vi "LDA_High_Convert_New.vi"(1 "dimensions":enum16{"1D", "2D"}(ring)=enum."2D", 2 "Create Sync Index":bool) -> (3 "LDA data":dbl[][](array[numeric]) format="%.3f", 5 "Diagnostic info":string[][](table), 6 "Sync Index":i32[](array[numeric]))   [LabVIEW 2017]
uses:
  BSA_Type.ctl
  Globals/LDA_meas_global_1.vi
  Globals/Plug_in_data_global.vi
  Globals/Meas_global.vi
  Globals/Preference_global.vi
  Globals/LDA_meas_global_2.vi
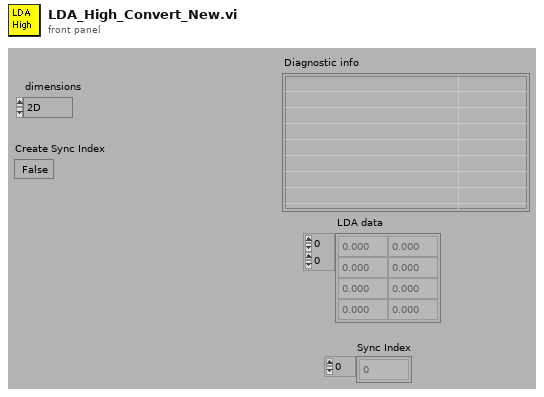
[diagram p1: front panel]
types:
  T1 = typedef "BSA_Type.ctl" = enum16{"57N11", "BSA F60"}
  T2 = enum16{"Velocity", "Transit time", "Arrival time"}[]
  T3 = typedef "Analysis_info_cluster.ctl" = cluster{"Colour":u32, "Inst type":T4, "Inst name":string, "Symbol":string, "Code name":string, "Extra Info":string, "Inst Array":T5, "Extra Titles":string[], "Extra Values":string[], "U":dbl, "u^2":dbl, "u^3":dbl, "u^4":dbl, "Skew_u":dbl, "Kurt_u":dbl, "Sd Error in Mean":dbl, "% u'/U":dbl, "X":dbl, "Y":dbl, "Z":dbl, "Timescale integral Estimate":dbl, "Sd Error in Variance":dbl, "Calib File":path, "Calib Constants":dbl[], "Output Position":bool, "Full Stats":bool, "Av Sampling Rate":dbl, "Av No of Samples":dbl, "Total Meas Time (s)":dbl, "ADAM Ch Name":string, "Max value":dbl, "Min value":dbl, "Sync Delay Time (s)":dbl, "Device ID":string, "Req Sample Rate Hz":dbl}
  T4 = typedef "Inst_type.ctl" = enum16{"Propeller anemometer", "Raw voltage", "Pressure Transducer", "Pitot-static tube", "Preston tube", "Hot wire", "Cross wire 1", "Cross wire 2", "Generic Linear", "Generic Polynomial", "Generic BackPoly", "Fast FID", "Thermocouple", "Cold wire", "Pulsed Wire", "LDA Vel", "LDA Tran time", "LDA Arr time", "Microphone"}
  T5 = typedef "Instrument_Array.ctl" = enum16{"PWA", "LDA", "Analogue"}
  T6 = typedef "Time_Trace_Cluster.ctl" = cluster{"Weighting":dbl[], "Time (s)":dbl[], "Voltage":dbl[], "Eng Values":dbl[]}
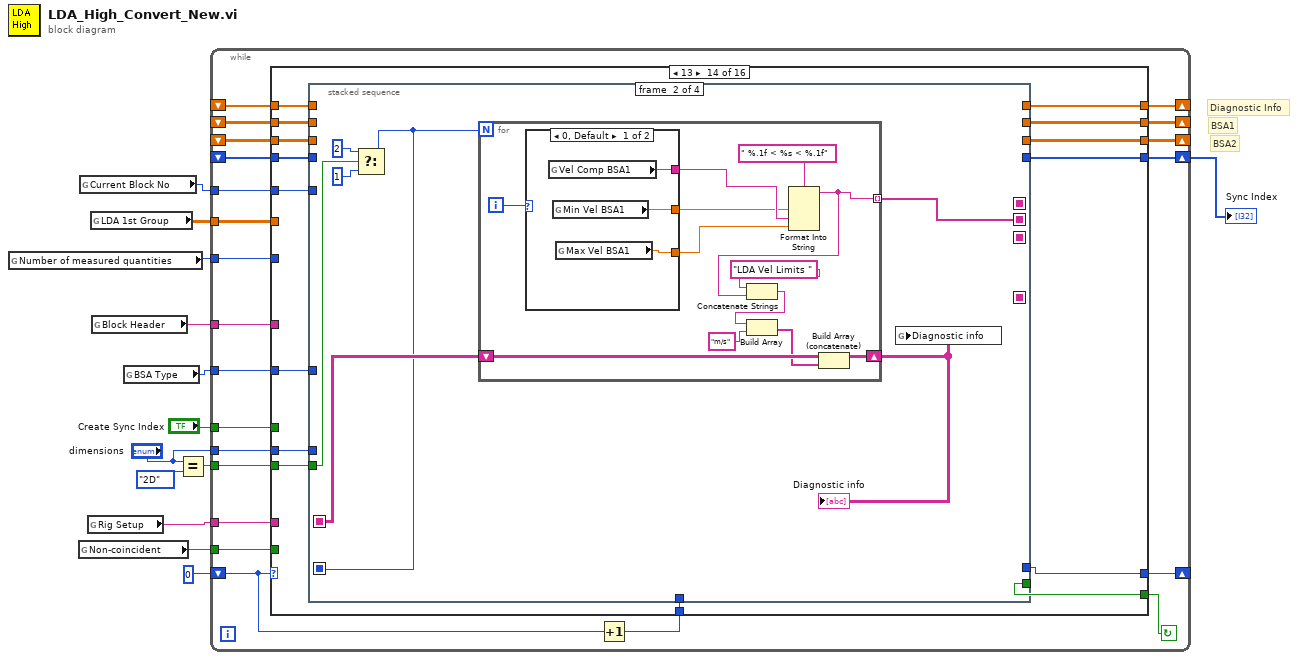
[diagram p0: block diagram]
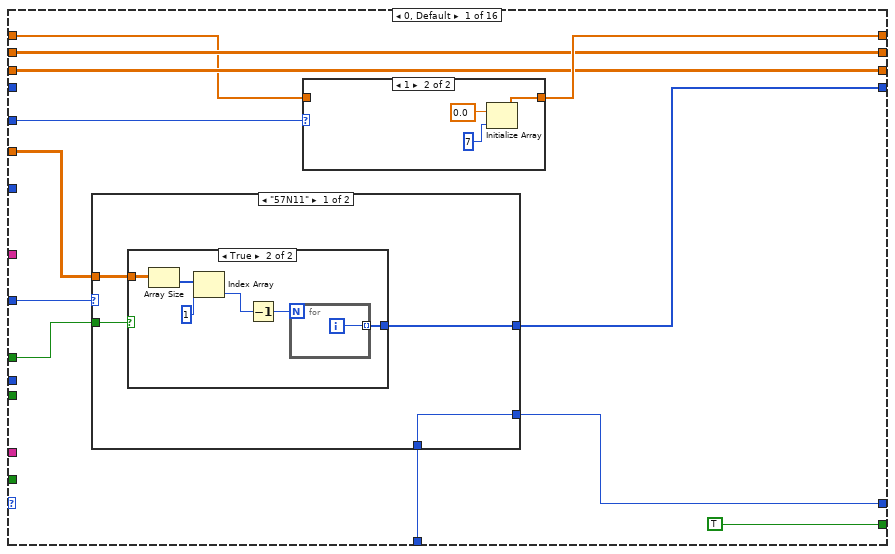
[diagram p2: hidden frame]
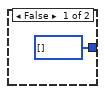
[diagram p4: hidden frame]
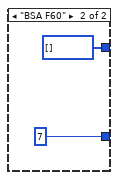
[diagram p5: hidden frame]
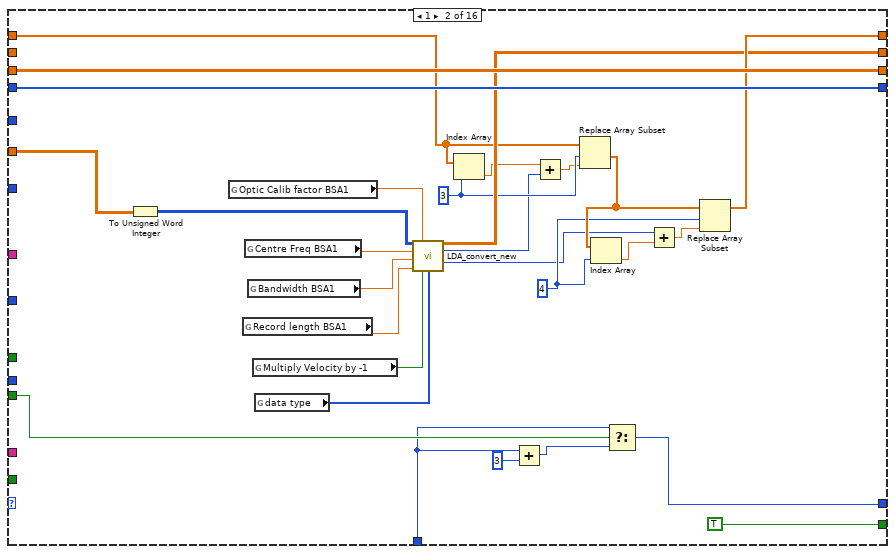
[diagram p6: hidden frame]
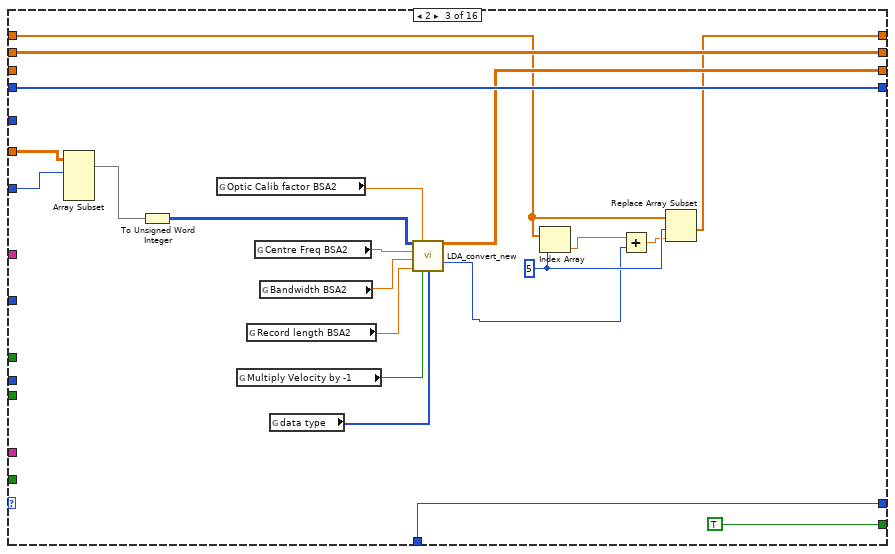
[diagram p7: hidden frame]
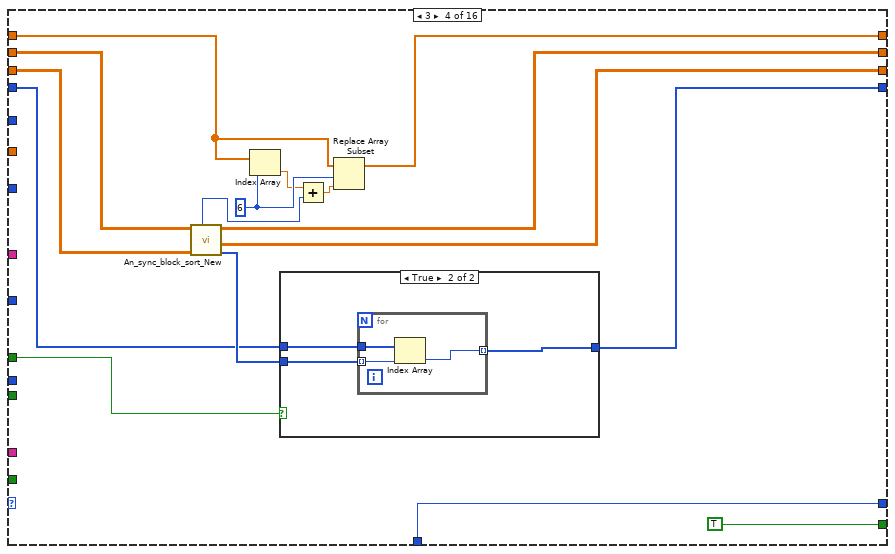
[diagram p8: hidden frame]
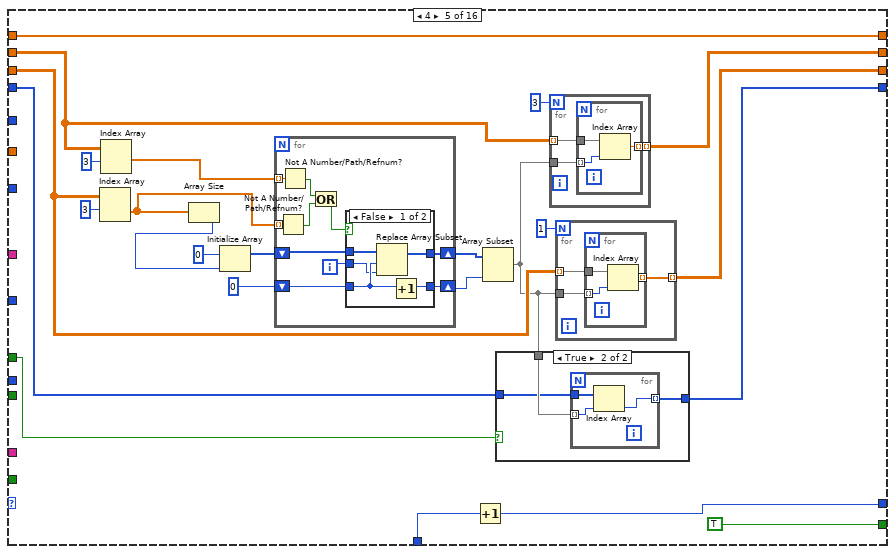
[diagram p10: hidden frame]
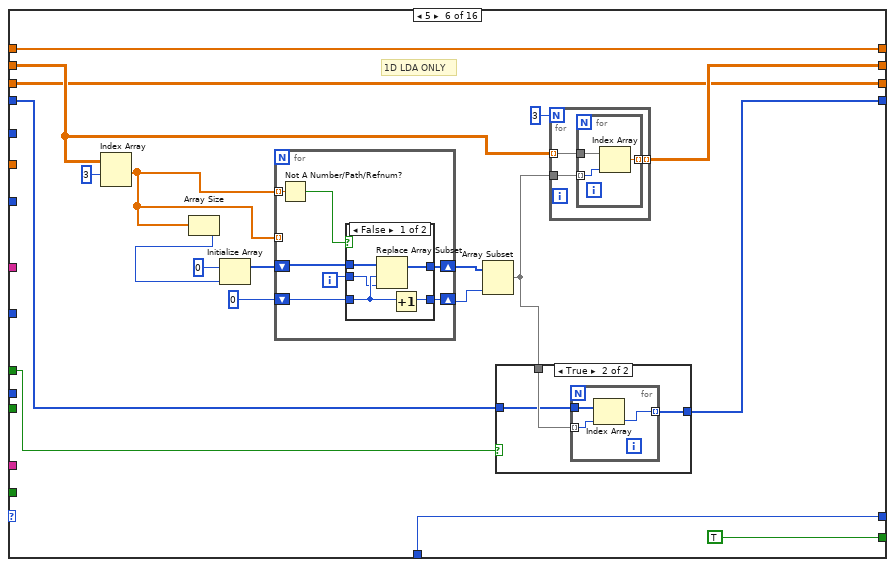
[diagram p13: hidden frame]
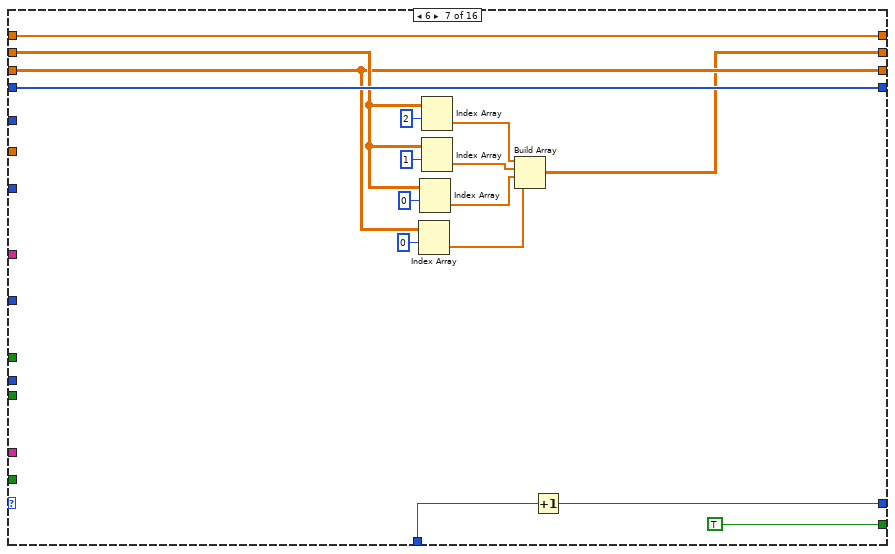
[diagram p16: hidden frame]
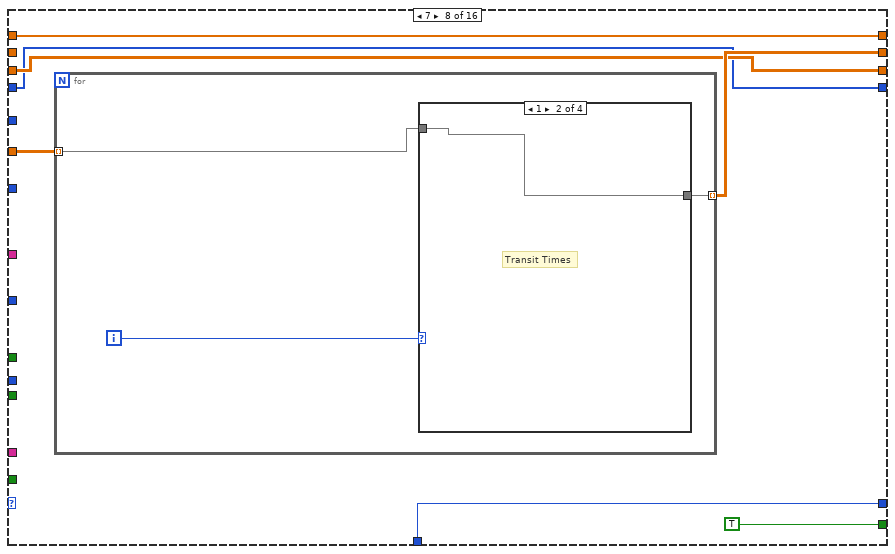
[diagram p17: hidden frame]
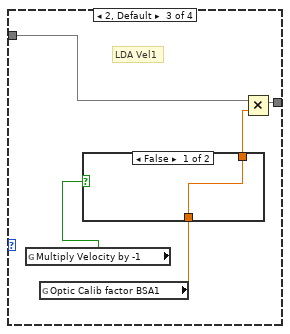
[diagram p19: hidden frame]
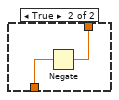
[diagram p20: hidden frame]
diagram:
  # "BSA2"
  # "BSA1"
  # "Diagnostic Info"
  n1 = global read "LDA_meas_global_1.vi" "Number of measured quantities"() -> (w9:i32)
  n2 = global read "LDA_meas_global_1.vi" "Non-coincident"() -> (w4:bool)
  n3 = global read "Meas_global.vi" "Current Block No"() -> (w5:i32)
  n4 = global read "Preference_global.vi" "Rig Setup"() -> (w3:string)
  n5 = global read "LDA_meas_global_2.vi" "LDA 1st Group"() -> (w1:dbl[][])
  n6 = global read "Plug_in_data_global.vi" "Block Header"() -> (w6:string)
  n7 = global read "LDA_meas_global_1.vi" "BSA Type"() -> (w2:T1)
  n8 = Equal?(x="dimensions", y=enum16{"1D", "2D"}."2D" ("dimensions")) -> (x = y?=w10:bool)
  n9 = while {
    tunnel: "dimensions" -> [w21]
    tunnel: w9 -> [w22]
    tunnel: w10 -> [w23]
    tunnel: "Create Sync Index" -> [w30]
    shift-left: _ -> [w24]
    shift-right: [w31] -> w7
    shift-left: _ -> [w27]
    shift-right: [w26] -> _
    shift-left: _ -> [w29]
    shift-right: [w28] -> _
    shift-left: _ -> [w25]
    shift-right: [w32] -> _
    shift-left: 0 -> [w34]
    shift-right: [w20] -> _
    tunnel: w2 -> [w19]
    tunnel: w6 -> [w18]
    tunnel: w5 -> [w17]
    tunnel: w4 -> [w16]
    tunnel: w3 -> [w15]
    tunnel: w1 -> [w14]
    stop <- w35 continue-if-true
    n10 = Increment(x=w34) -> (x+1=w33:i32)
    n11 = case shown="13" w34 {
      tunnel: [TRUE TRUE TRUE TRUE TRUE TRUE TRUE TRUE TRUE TRUE TRUE TRUE TRUE w410 w538 FALSE] -> w35
      tunnel: w33 -> [w39 w82 w105 w129 w139 w215 w258 w262 w306 w315 w339 w367 w388 w409 w546 w606]
      tunnel: [w46 w86 w98 w124 w140 w200 w244 w263 w297 w314 w348 w368 w387 w418 w543 w604] -> w32
      tunnel: [w45 w91 w113 w120 w145 w202 w257 w264 w308 w316 w347 w369 w389 w411 w544 w608] -> w31
      tunnel: w30 -> [w44 _ _ w123 w147 w204 _ _ _ _ _ _ _ _ _ _]
      tunnel: w29 -> [w43 _ w112 w128 w149 w206 w249 _ w292 w312 w343 w364 w385 w416 w534 w590]
      tunnel: [w43 w85 w112 w126 w148 w205 w247 w266 w292 w311 w343 w364 w385 w415 w534 w590] -> w28
      tunnel: w27 -> [w42 w92 _ w127 w144 w198 w248 w265 w307 w310 w346 _ w384 w413 w545 w607]
      tunnel: [w42 w92 w111 w125 w143 w198 w248 w265 w307 w310 w346 w363 w383 w414 w545 w607] -> w26
      tunnel: w25 -> [w38 w77 w99 w118 w140 w200 w244 w263 w298 w314 w348 w368 w387 w417 w543 w604]
      tunnel: w24 -> [_ w91 w113 w121 w146 w203 w257 w264 w308 w316 w347 w369 w389 w412 w544 w608]
      tunnel: w23 -> [_ w84 _ _ _ _ _ _ _ _ _ _ _ w405 _ _]
      tunnel: w22 -> [_ _ w110 _ _ _ _ _ _ _ _ _ _ _ _ _]
      tunnel: w21 -> [_ _ _ _ _ _ _ _ _ _ w344 _ _ w407 _ _]
      tunnel: [w40 w83 w105 w129 w138 w215 w246 w262 w306 w315 w337 w367 w388 w404 w546 w606] -> w20
      tunnel: w19 -> [w41 _ _ _ _ _ _ _ _ w313 _ _ w386 w408 w541 _]
      tunnel: w18 -> [_ _ _ _ _ _ _ _ _ _ _ _ _ _ _ _]
      tunnel: w17 -> [w37 _ _ _ _ _ _ _ _ _ _ _ _ w406 w531 w592]
      tunnel: w16 -> [_ _ _ _ _ _ _ _ _ _ w341 _ _ _ w535 _]
      tunnel: w15 -> [_ _ _ _ _ _ _ _ _ _ _ _ _ _ _ _]
      tunnel: w14 -> [w36 w67 w96 _ _ _ _ w260 _ _ _ _ _ _ _ _]
      frame 0, Default {
        n12 = case shown="\"57N11\"" w41 {
          tunnel: [w55 i32[] []] -> w45
          tunnel: w44 -> [w54 _]
          tunnel: w36 -> [w53 _]
          tunnel: [w52 7] -> w40
          tunnel: w39 -> [w52 _]
          frame "57N11" {
            n13 = case shown="True" w54 {
              tunnel: [i32[] [] w62] -> w55
              tunnel: w53 -> [_ w61]
              frame False {
              }
              frame True {
                n14 = Array Size(array=w61) -> (size(s)=w60:i32[])
                n15 = Index Array(array=w60, index=1 ("Index")) -> (element=w59:i32)
                n16 = Decrement(x=w59) -> (x-1=w58:i32)
                n17 = for {
                  N: w58 -> [_]
                  tunnel: [w63] -> w62 mode=indexing
                  i -> [w63]
                }
              }
            }
          }
          frame "BSA F60" {
          }
        }
        n18 = case shown="1" w37 {
          tunnel: [w48 w49] -> w46
          tunnel: w38 -> [w48 _]
          frame 2, Default {
          }
          frame 1 {
            n19 = Initialize Array(0.0, 7 ("Dimension Size")) -> (w49:dbl[])
          }
        }
      }
      frame 1 {
        w71 = 4 ("Index")
        w76 = 3 ("Index")
        n20 = To Unsigned Word Integer(number=w67) -> (unsigned 16bit integer=w66:u16[][])
        n21 = global read "LDA_meas_global_1.vi" "Optic Calib factor BSA1"() -> (w78:dbl)
        n22 = global read "LDA_meas_global_1.vi" "Record length BSA1"() -> (w88:dbl)
        n23 = global read "LDA_meas_global_1.vi" "Centre Freq BSA1"() -> (w90:dbl)
        n24 = global read "LDA_meas_global_1.vi" "Bandwidth BSA1"() -> (w89:dbl)
        n25 = global read "LDA_meas_global_1.vi" "Multiply Velocity by -1"() -> (w79:bool)
        n26 = global read "LDA_meas_global_1.vi" "data type"() -> (w87:T2)
        n27 = call "LDA_convert_new.vi"("binary data"=w66, "Calibration factor"=w78, "Centre frequency"=w90, "Bandwidth"=w89, "Record length (RL)"=w88, "Multiply Velocity by -1"=w79, "data type"=w87) -> ("Converted results"=w85:dbl[][], "No of cntr resets"=w74:i32, "No invalid"=w69:i32)  [unwired: 1 in, 5 out]
        n28 = Index Array(array=w77, index=w76) -> (element=w75:dbl)
        n29 = Add(x=w82, y=3) -> (x+y=w80:i32)
        n30 = Add(x=w75, y=w74) -> (x+y=w73:dbl)
        n31 = Replace Array Subset(array=w77, new element=w73, index=w76) -> (w72:dbl[])
        n32 = Index Array(array=w72, index=w71) -> (element=w68:dbl)
        n33 = Select(t=w82, s=w84, f=w80) -> (s? t:f=w83:i32)
        n34 = Add(x=w69, y=w68) -> (x+y=w70:dbl)
        n35 = Replace Array Subset(array=w72, new element=w70, index=w71) -> (w86:dbl[])
      }
      frame 2 {
        w102 = 5 ("Index")
        n36 = Array Subset(array=w96, index (row)=w110) -> (w95:dbl[][])  [unwired: 3 in]
        n37 = To Unsigned Word Integer(number=w95) -> (unsigned 16bit integer=w94:u16[][])
        n38 = global read "LDA_meas_global_2.vi" "Optic Calib factor BSA2"() -> (w103:dbl)
        n39 = global read "LDA_meas_global_2.vi" "Multiply Velocity by -1"() -> (w104:bool)
        n40 = global read "LDA_meas_global_2.vi" "Record length BSA2"() -> (w108:dbl)
        n41 = global read "LDA_meas_global_2.vi" "Centre Freq BSA2"() -> (w106:dbl)
        n42 = global read "LDA_meas_global_2.vi" "Bandwidth BSA2"() -> (w107:dbl)
        n43 = global read "LDA_meas_global_2.vi" "data type"() -> (w109:T2)
        n44 = call "LDA_convert_new.vi"("binary data"=w94, "Calibration factor"=w103, "Centre frequency"=w106, "Bandwidth"=w107, "Record length (RL)"=w108, "Multiply Velocity by -1"=w104, "data type"=w109) -> ("Converted results"=w111:dbl[][], "No invalid"=w97:i32)  [unwired: 1 in, 6 out]
        n45 = Index Array(array=w99, index=w102) -> (element=w101:dbl)
        n46 = Add(x=w101, y=w97) -> (x+y=w100:dbl)
        n47 = Replace Array Subset(array=w99, new element=w100, index=w102) -> (w98:dbl[])
      }
      frame 3 {
        w119 = 6 ("Index")
        n48 = call "An_sync_block_sort_New.vi"("BSA 2"=w127, "BSA 1"=w128) -> ("Analogue Sync Index"=w122:i32[], "BSA 2 Sync"=w125:dbl[][], "BSA 1 Sync"=w126:dbl[][], "No of slips"=w115:i32)  [unwired: 4 out]
        n49 = Index Array(array=w118, index=w119) -> (element=w116:dbl)
        n50 = case shown="True" w123 {
          tunnel: w122 -> [_ w134]
          tunnel: w121 -> [w131 w133]
          tunnel: [w131 w132] -> w120
          frame False {
          }
          frame True {
            n51 = for {
              tunnel: w134 -> [w137] mode=indexing
              tunnel: w133 -> [w136]
              tunnel: [w135] -> w132 mode=indexing
              n52 = Index Array(array=w136, index=w137) -> (element=w135:i32)
            }
          }
        }
        n53 = Add(x=w116, y=w115) -> (x+y=w117:dbl)
        n54 = Replace Array Subset(array=w118, new element=w117, index=w119) -> (w124:dbl[])
      }
      frame 4 {
        n55 = Index Array(array=w144, index (row)=3 ("Index")) -> (element=w152:dbl[])  [unwired: 1 in]
        n56 = Index Array(array=w149, index (row)=3 ("Index")) -> (element=w151:dbl[])  [unwired: 1 in]
        n57 = Array Size(array=w152) -> (size(s)=w154:i32)
        n58 = Initialize Array(0, w154) -> (w156:i32[])
        n59 = for {
          shift-right: [w189] -> w158
          shift-left: w156 -> [w190]
          shift-right: [w187] -> w153
          shift-left: 0 -> [w188]
          tunnel: w152 -> [w183] mode=indexing
          tunnel: w151 -> [w182] mode=indexing
          i -> [w186]
          n60 = Not A Number/Path/Refnum?(number/path/refnum=w183) -> (NaN/Path/Refnum?=w185:bool)
          n61 = Not A Number/Path/Refnum?(number/path/refnum=w182) -> (NaN/Path/Refnum?=w184:bool)
          n62 = Or(x=w184, y=w185) -> (x .or. y?=w181:bool)
          n63 = case shown="False" w181 {
            tunnel: w190 -> [w195 w197]
            tunnel: [w194 w197] -> w189
            tunnel: w188 -> [w193 w196]
            tunnel: [w192 w196] -> w187
            tunnel: w186 -> [w191 _]
            frame False {
              n64 = Replace Array Subset(array=w195, new element=w191, index=w193) -> (w194:i32[])
              n65 = Increment(x=w193) -> (x+1=w192:i32)
            }
            frame True {
            }
          }
        }
        n66 = Increment(x=w139) -> (x+1=w138:i32)
        n67 = Array Subset(array=w158, length=w153) -> (w141:i32[])  [unwired: 1 in]
        n68 = case shown="True" w147 {
          tunnel: w141 -> [_ w171]
          tunnel: w146 -> [w168 w170]
          tunnel: [w168 w169] -> w145
          frame False {
          }
          frame True {
            n69 = for {
              tunnel: w171 -> [w173] mode=indexing
              tunnel: w170 -> [w174]
              tunnel: [w172] -> w169 mode=indexing
              n70 = Index Array(array=w174, index=w173) -> (element=w172:i32)
            }
          }
        }
        n71 = for {
          N: 3 -> [_]
          tunnel: w149 -> [w177] mode=indexing
          tunnel: w141 -> [w176]
          tunnel: [w175] -> w148 mode=indexing
          n72 = for {
            tunnel: w176 -> [w179] mode=indexing
            tunnel: w177 -> [w180]
            tunnel: [w178] -> w175 mode=indexing
            n73 = Index Array(array=w180, index=w179) -> (element=w178:dbl)
          }
        }
        n74 = for {
          N: 1 -> [_]
          tunnel: w141 -> [w164]
          tunnel: w144 -> [w163] mode=indexing
          tunnel: [w162] -> w143 mode=indexing
          n75 = for {
            tunnel: w164 -> [w166] mode=indexing
            tunnel: w163 -> [w167]
            tunnel: [w165] -> w162 mode=indexing
            n76 = Index Array(array=w167, index=w166) -> (element=w165:dbl)
          }
        }
      }
      frame 5 {
        # "1D LDA ONLY"
        n77 = Index Array(array=w206, index (row)=3 ("Index")) -> (element=w199:dbl[])  [unwired: 1 in]
        n78 = Array Size(array=w199) -> (size(s)=w209:i32)
        n79 = Initialize Array(0, w209) -> (w211:i32[])
        n80 = for {
          shift-right: [w235] -> w213
          shift-left: w211 -> [w236]
          shift-right: [w233] -> w208
          shift-left: 0 -> [w234]
          tunnel: w199 -> [_] mode=indexing
          tunnel: w199 -> [w231] mode=indexing
          i -> [w232]
          n81 = Not A Number/Path/Refnum?(number/path/refnum=w231) -> (NaN/Path/Refnum?=w230:bool)
          n82 = case shown="False" w230 {
            tunnel: w236 -> [w241 w243]
            tunnel: [w240 w243] -> w235
            tunnel: w234 -> [w239 w242]
            tunnel: [w238 w242] -> w233
            tunnel: w232 -> [w237 _]
            frame False {
              n83 = Replace Array Subset(array=w241, new element=w237, index=w239) -> (w240:i32[])
              n84 = Increment(x=w239) -> (x+1=w238:i32)
            }
            frame True {
            }
          }
        }
        n85 = Array Subset(array=w213, length=w208) -> (w201:i32[])  [unwired: 1 in]
        n86 = case shown="True" w204 {
          tunnel: w201 -> [_ w220]
          tunnel: w203 -> [w217 w219]
          tunnel: [w217 w218] -> w202
          frame False {
          }
          frame True {
            n87 = for {
              tunnel: w220 -> [w222] mode=indexing
              tunnel: w219 -> [w223]
              tunnel: [w221] -> w218 mode=indexing
              n88 = Index Array(array=w223, index=w222) -> (element=w221:i32)
            }
          }
        }
        n89 = for {
          N: 3 -> [_]
          tunnel: w206 -> [w226] mode=indexing
          tunnel: w201 -> [w225]
          tunnel: [w224] -> w205 mode=indexing
          n90 = for {
            tunnel: w225 -> [w228] mode=indexing
            tunnel: w226 -> [w229]
            tunnel: [w227] -> w224 mode=indexing
            n91 = Index Array(array=w229, index=w228) -> (element=w227:dbl)
          }
        }
      }
      frame 6 {
        n92 = Index Array(array=w248, index (row)=0) -> (element=w245:dbl[])  [unwired: 1 in]
        n93 = Index Array(array=w249, index (row)=0) -> (element=w250:dbl[])  [unwired: 1 in]
        n94 = Index Array(array=w249, index (row)=2) -> (element=w252:dbl[])  [unwired: 1 in]
        n95 = Index Array(array=w249, index (row)=1) -> (element=w251:dbl[])  [unwired: 1 in]
        n96 = Build Array(w252, w251, w250, w245) -> (w247:dbl[][])
        n97 = Increment(x=w258) -> (x+1=w246:i32)
      }
      frame 7 {
        n98 = for {
          tunnel: [w268] -> w266 mode=indexing
          tunnel: w260 -> [w267] mode=indexing
          i -> [w269]
          n99 = case shown="1" w269 {
            tunnel: w267 -> [w270 w271 w276 w284]
            tunnel: [w270 w271 w275 w283] -> w268
            frame 0 {
              # "Arrival Times"
            }
            frame 1 {
              # "Transit Times"
            }
            frame 2, Default {
              # "LDA Vel1"
              n100 = global read "LDA_meas_global_1.vi" "Multiply Velocity by -1"() -> (w274:bool)
              n101 = global read "LDA_meas_global_1.vi" "Optic Calib factor BSA1"() -> (w273:dbl)
              n102 = case shown="False" w274 {
                tunnel: w273 -> [w277 w279]
                tunnel: [w277 w278] -> w272
                frame False {
                }
                frame True {
                  n103 = Negate(x=w279) -> (-x=w278:dbl)
                }
              }
              n104 = Multiply(x=w276, y=w272) -> (x*y=w275:dbl[])
            }
            frame 3 {
              # "LDA Vel2"
              n105 = global read "LDA_meas_global_2.vi" "Multiply Velocity by -1"() -> (w282:bool)
              n106 = global read "LDA_meas_global_2.vi" "Optic Calib factor BSA2"() -> (w281:dbl)
              n107 = case shown="True" w282 {
                tunnel: w281 -> [w285 w287]
                tunnel: [w285 w286] -> w280
                frame False {
                }
                frame True {
                  n108 = Negate(x=w287) -> (-x=w286:dbl)
                }
              }
              n109 = Multiply(x=w284, y=w280) -> (x*y=w283:dbl[])
            }
          }
        }
      }
      frame 8 {
        w301 = 1 ("Index")
        w303 = 0 ("Index")
        n110 = Index Array(array=w292, index (row)=0 ("Index")) -> (element=w289:dbl[])  [unwired: 1 in]
        n111 = Array Size(array=w289) -> (size(s)=w290:i32)
        n112 = Decrement(x=w290) -> (x-1=w291:i32)
        n113 = Array Size(array=w292) -> (size(s)=w305:i32[])
        n114 = Index Array(array=w289, index=w291) -> (element=w288:dbl)
        n115 = global write "LDA_meas_global_1.vi" "Time for last Block (s)"(w288) -> ()
        n116 = Index Array(array=w298, index=w303) -> (element=w302:dbl)
        n117 = Index Array(array=w305, index=1 ("Index")) -> (element=w296:i32)
        n118 = Add(x=w302, y=w288) -> (x+y=w294:dbl)
        n119 = Replace Array Subset(array=w298, new element=w294, index=w303) -> (w299:dbl[])
        n120 = Index Array(array=w299, index=w301) -> (element=w300:dbl)
        n121 = Add(x=w300, y=w296) -> (x+y=w295:dbl)
        n122 = Replace Array Subset(array=w299, new element=w295, index=w301) -> (w297:dbl[])
      }
      frame 9 {
        n123 = for {
          tunnel: w312 -> [w320] mode=indexing
          tunnel: [w319] -> w311 mode=indexing
          tunnel: w313 -> [w318]
          i -> [w321]
          n124 = case shown="0" w321 {
            tunnel: w320 -> [w323 w329 w336]
            tunnel: [w323 w330 w336] -> w319
            tunnel: w318 -> [w324 w331 _]
            frame 0 {
              n125 = case shown="\"57N11\"" w324 {
                tunnel: [w325 w328] -> w322
                tunnel: w323 -> [w327 w328]
                frame "57N11" {
                  n126 = Multiply(x=0.001, y=w327) -> (x*y=w325:dbl[])
                }
                frame "BSA F60" {
                }
              }
              n127 = global write "LDA_meas_global_1.vi" "Arrival times"(w322) -> ()
            }
            frame 1 {
              # "Transit Times"
              n128 = case shown="\"57N11\"" w331 {
                tunnel: [w332 w333] -> w330
                tunnel: w329 -> [w332 w335]
                frame "57N11" {
                }
                frame "BSA F60" {
                  n129 = Multiply(x=1000000.0, y=w335) -> (x*y=w333:dbl[])
                }
              }
              n130 = global write "LDA_meas_global_1.vi" "Transit times"(w330) -> ()
            }
            frame 2, Default {
              # "LDA Vel2"
              # "LDA Vel1"
            }
          }
        }
      }
      frame 10 {
        n131 = case shown="\"2D\"" w344 {
          tunnel: [w353 w356] -> w345
          tunnel: w341 -> [_ w355]
          frame "1D" {
            n132 = Build Array(2) -> (w353:i32[])
          }
          frame "2D" {
            n133 = case shown="True" w355 {
              tunnel: [w358 w360] -> w356
              frame True {
                n134 = Build Array(2, 2) -> (w358:i32[])
              }
              frame False {
                n135 = Build Array(2, 3 ("element")) -> (w360:i32[])
              }
            }
          }
        }
        n136 = Increment(x=w339) -> (x+1=w340:i32)
        n137 = Increment(x=w340) -> (x+1=w338:i32)
        n138 = for {
          tunnel: w343 -> [w352]
          tunnel: w345 -> [w351] mode=indexing
          tunnel: [w350] -> w342 mode=indexing
          n139 = Index Array(array=w352, index (row)=w351) -> (element=w350:dbl[])  [unwired: 1 in]
        }
        "LDA data" <- w342
        n140 = Select(t=w339, s=w341, f=w338) -> (s? t:f=w337:i32)
      }
      frame 11 {
        n141 = global read "LDA_meas_global_2.vi" "LDA 2nd Group"() -> (w365:dbl[][])
        n142 = for {
          tunnel: [w371] -> w363 mode=indexing
          tunnel: w365 -> [w370] mode=indexing
          i -> [w372]
          n143 = case shown="0" w372 {
            tunnel: w370 -> [w373 w374 w379]
            tunnel: [w373 w374 w378] -> w371
            frame 0 {
              # "Arrival Times"
            }
            frame 1 {
              # "Transit Times"
            }
            frame 2, Default {
              # "LDA Vel2"
              n144 = global read "LDA_meas_global_2.vi" "Multiply Velocity by -1"() -> (w377:bool)
              n145 = global read "LDA_meas_global_2.vi" "Optic Calib factor BSA2"() -> (w376:dbl)
              n146 = case shown="True" w377 {
                tunnel: w376 -> [w380 w382]
                tunnel: [w380 w381] -> w375
                frame False {
                }
                frame True {
                  n147 = Negate(x=w382) -> (-x=w381:dbl)
                }
              }
              n148 = Multiply(x=w379, y=w375) -> (x*y=w378:dbl[])
            }
          }
        }
      }
      frame 12 {
        n149 = for {
          tunnel: w384 -> [w393] mode=indexing
          tunnel: [w392] -> w383 mode=indexing
          tunnel: w386 -> [w391]
          i -> [w394]
          n150 = case shown="0" w394 {
            tunnel: w393 -> [w395 w397 w403]
            tunnel: [w395 w396 w403] -> w392
            tunnel: w391 -> [_ w398 _]
            frame 0 {
              # "Arrival Times"
              n151 = global write "LDA_meas_global_2.vi" "Arrival times LDA2"(w395) -> ()
            }
            frame 1 {
              # "Transit Times"
              n152 = case shown="\"BSA F60\"" w398 {
                tunnel: [w399 w400] -> w396
                tunnel: w397 -> [w399 w402]
                frame "57N11" {
                }
                frame "BSA F60" {
                  n153 = Multiply(x=1000000.0, y=w402) -> (x*y=w400:dbl[])
                }
              }
              n154 = global write "LDA_meas_global_2.vi" "Transit times LDA2"(w396) -> ()
            }
            frame 2, Default {
              # "LDA Vel2"
              # "LDA Vel1"
              n155 = global write "LDA_meas_global_2.vi" "Vel LDA2 Non Coincident"(w403) -> ()
            }
          }
        }
      }
      frame 13 {
        n156 = stacked-sequence {
          seq-local: [w423 _ _ _] -> [_ _ _ w512]
          seq-local: [w424 _ _ _] -> [_ _ _ w502]
          seq-local: [_ w459 _ _] -> [_ _ _ w511]
          seq-local: [w422 _ _ _] -> [_ w458 _ _]
          seq-local: [_ w456 _ _] -> [_ _ w487 _]
          seq-local: [_ _ w481 _] -> [_ _ _ w508]
          tunnel: [w421 _ _ _] -> w418
          tunnel: w417 -> [w421 _ _ _]
          tunnel: w416 -> [_ _ _ w516]
          tunnel: [_ _ _ w516] -> w415
          tunnel: [_ _ _ w515] -> w414
          tunnel: w413 -> [_ _ _ w515]
          tunnel: w412 -> [_ _ _ w514]
          tunnel: [_ _ _ w514] -> w411
          tunnel: [TRUE _ _ _] -> w410
          tunnel: w409 -> [w430 _ _ _]
          tunnel: [w430 _ _ _] -> w404
          tunnel: w408 -> [w435 _ _ _]
          tunnel: w407 -> [w427 _ _ _]
          tunnel: w406 -> [w429 _ _ _]
          tunnel: w405 -> [_ w460 _ w509]
          frame #0 {
            n157 = Divide(x=w421, y=w429) -> (x/y=w419:dbl[])
            n158 = case shown="\"BSA F60\"" w435 {
              tunnel: w427 -> [w446 _]
              tunnel: "No of:Resets::" -> [w445 _]
              tunnel: "No of:Invalid:Bursts BSA 1:" -> [w444 _]
              tunnel: "No of:invalid:Bursts BSA 2:" -> [w443 _]
              tunnel: "No of:Slips:in Arrival:times" -> [w442 _]
              tunnel: w429 -> [w441 _]
              tunnel: [w440 string[] []] -> w424
              frame "57N11" {
                n159 = case shown="\"2D\"" w446 {
                  tunnel: w445 -> [w451 w454]
                  tunnel: w444 -> [w450 w453]
                  tunnel: w443 -> [w449 _]
                  tunnel: w442 -> [w448 _]
                  tunnel: w441 -> [_ _]
                  tunnel: [w447 w452] -> w440
                  frame "2D" {
                    n160 = Build Array(w451, w450, w449, w448) -> (w447:string[])
                  }
                  frame "1D" {
                    n161 = Build Array(w454, w453) -> (w452:string[])
                  }
                }
              }
              frame "BSA F60" {
              }
            }
            n162 = Array Size(array=w424) -> (size(s)=w428:i32)
            n163 = Array Subset(array=w419, index=3, length=w428) -> (w426:dbl[])
            n164 = Number To Fractional String(number=w426, precision (6)=i16 2) -> (F-format string=w423:string[])  [unwired: 2 out]
            n165 = for {
              tunnel: w424 -> [w439] mode=indexing
              tunnel: w423 -> [w438] mode=indexing
              tunnel: [w437] -> w422 mode=indexing
              n166 = Build Array(w439, w438) -> (w437:string[])
            }
          }
          frame #1 {
            n167 = Select(t=2, s=w460, f=1) -> (s? t:f=w456:i32)
            n168 = for {
              N: w456 -> [_]
              shift-right: [w472] -> w457
              shift-left: w458 -> [w473]
              tunnel: [w463] -> w459 mode=indexing
              i -> [w474]
              n169 = case shown="0, Default" w474 {
                tunnel: [w477 w480] -> w468
                tunnel: [w476 w479] -> w467
                tunnel: [w475 w478] -> w466
                frame 0, Default {
                  n170 = global read "LDA_meas_global_1.vi" "Vel Comp BSA1"() -> (w477:string)
                  n171 = global read "LDA_meas_global_1.vi" "Min Vel BSA1"() -> (w476:dbl)
                  n172 = global read "LDA_meas_global_1.vi" "Max Vel BSA1"() -> (w475:dbl)
                }
                frame 1 {
                  n173 = global read "LDA_meas_global_2.vi" "Vel Comp BSA2"() -> (w480:string)
                  n174 = global read "LDA_meas_global_2.vi" "Max Vel BSA2"() -> (w478:dbl)
                  n175 = global read "LDA_meas_global_2.vi" "Min Vel BSA2"() -> (w479:dbl)
                }
              }
              n176 = Format Into String(format string=" %.1f < %s < %.1f" ("Format String"), w467, w468, w466) -> (resulting string=w463:string)  [unwired: 2 in, 1 out]
              n177 = Concatenate Strings("LDA Vel Limits " ("element"), w463) -> (w464:string)
              n178 = Build Array(w464, "m/s" ("Input Element")) -> (w469:string[])
              n179 = Build Array (concatenate)(w473, w469) -> (w472:string[][])
            }
            "Diagnostic info" <- w457
            n180 = global write "Meas_global.vi" "Diagnostic info"(w457) -> ()
          }
          frame #2 {
            n181 = for {
              N: w487 -> [_]
              tunnel: [w489] -> w482 mode=concatenating
              i -> [w494]
              n182 = case shown="1" w494 {
                tunnel: [w497 w500] -> w493
                tunnel: [w496 w499] -> w492
                tunnel: [w495 w498] -> w488
                frame 0, Default {
                  n183 = global read "LDA_meas_global_1.vi" "Beam Separation (mm)"() -> (w496:dbl)
                  n184 = global read "LDA_meas_global_1.vi" "Focal Length (mm)"() -> (w497:dbl)
                  n185 = global read "LDA_meas_global_1.vi" "Probe Type"() -> (w495:string)
                }
                frame 1 {
                  n186 = global read "LDA_meas_global_2.vi" "Beam Separation 2 (mm)"() -> (w499:dbl)
                  n187 = global read "LDA_meas_global_2.vi" "Focal Length 2 (mm)"() -> (w500:dbl)
                  n188 = global read "LDA_meas_global_2.vi" "Probe Type 2"() -> (w498:string)
                }
              }
              n189 = call "Number_2_string.vi"("number"=w493) -> ("String"=w490:string)  [unwired: 1 in]
              n190 = call "Number_2_string.vi"("number"=w492) -> ("String"=w491:string)  [unwired: 1 in]
              n191 = Build Array(w488, w490, w491) -> (w489:string[])
            }
            n192 = global read "LDA_meas_global_1.vi" "Using 45 Degree Mirror?"() -> (w486:bool)
            n193 = Select(t="45 Deg Mirror", s=w486, f="None") -> (s? t:f=w483:string)
            n194 = Build Array (concatenate)(w482, w483) -> (w481:string[])
          }
          frame #3 {
            n195 = case shown="False" w509 {
              tunnel: "LDA:Vel Limits:BSA1" ("Input Element") -> [w525 w530]
              tunnel: [w524 w529] -> w505
              tunnel: "LDA:Focal Length:BSA1" ("Input Element") -> [w518 w528]
              tunnel: "LDA:Beam Separation:BSA1" ("Input Element") -> [w522 w527]
              tunnel: "LDA:Probe_Type:BSA1" ("Input Element") -> [w519 w526]
              frame True {
                n196 = Build Array(w525, "LDA:Vel Limits:BSA2" ("Input Element"), w519, w518, w522, "LDA:Probe_Type:BSA2" ("Input Element"), "LDA:Focal Length:BSA2" ("Input Element"), "LDA:Beam Separation:BSA2" ("Input Element")) -> (w524:string[])
              }
              frame False {
                n197 = Build Array(w530, w526, w528, w527) -> (w529:string[])
              }
            }
            n198 = Build Array (concatenate)(w512, w511, w508) -> (w510:string[])
            n199 = global write "LDA_meas_global_1.vi" "LDA Results file Values"(w510) -> ()
            n200 = Build Array (concatenate)(w502, w505, "LDA:45_Deg:Mirror" ("Input Element")) -> (w504:string[])
            n201 = global write "LDA_meas_global_1.vi" "LDA Results file headers"(w504) -> ()
          }
        }
      }
      frame 14 {
        n202 = global read "Meas_global.vi" "Processing last block?"() -> (w540:bool)
        n203 = global read "Meas_global.vi" "Analysis Info cluster"() -> (w537:T3[])
        n204 = Equal?(x=BSA_Type."57N11" ("BSA Type"), y=w541) -> (x = y?=w539:bool)
        n205 = global read "Meas_global.vi" "Time Trace"() -> (w533:T6[])
        n206 = for {
          tunnel: w537 -> [w552] mode=indexing
          tunnel: [w553] -> w536 mode=indexing
          tunnel: w535 -> [w551]
          tunnel: w534 -> [w550]
          tunnel: w533 -> [w549] mode=indexing
          tunnel: [w548] -> w532 mode=indexing
          tunnel: w531 -> [w547]
          n207 = Unbundle By Name(w552) -> ("Code name"=w554:string)
          n208 = case shown="\"2LDA:U\"" w554 {
            tunnel: [w556 w558 w569] -> w553
            tunnel: w552 -> [w556 w559 w570]
            tunnel: w551 -> [_ _ w578]
            tunnel: w550 -> [_ w565 w577]
            tunnel: w549 -> [w555 w562 w576]
            tunnel: [w555 w560 w571] -> w548
            tunnel: w547 -> [_ w557 w568]
            frame "False", Default {
            }
            frame "1LDA:U" {
              n209 = global read "LDA_meas_global_1.vi" "Arrival times"() -> (w567:dbl[])
              n210 = global read "LDA_meas_global_1.vi" "Transit times"() -> (w566:dbl[])
              n211 = Index Array(array=w565, index (row)=2) -> (element=w563:dbl[])  [unwired: 1 in]
              n212 = Bundle By Name(cluster=w562, "Eng Values"=w563, "Time (s)"=w567, "Weighting"=w566) -> (w561:T6)
              n213 = call "Remove_LDA_Spikes.vi"("Current Block Number"=w557, "Analaysis info Cluster"=w559, "Time Trace In"=w561) -> ("Analaysis info Cluster Out"=w558:T3, "Time trace Out"=w560:T6)  [unwired: 1 in]
            }
            frame "2LDA:U" {
              n214 = case shown="False" w578 {
                tunnel: [w583 w585] -> w573
                tunnel: [w582 w586] -> w575
                tunnel: [w579 w584] -> w574
                tunnel: w577 -> [w580 _]
                frame False {
                  n215 = global read "LDA_meas_global_1.vi" "Transit times"() -> (w582:dbl[])
                  n216 = global read "LDA_meas_global_1.vi" "Arrival times"() -> (w583:dbl[])
                  n217 = Index Array(array=w580, index (row)=3) -> (element=w579:dbl[])  [unwired: 1 in]
                }
                frame True {
                  n218 = global read "LDA_meas_global_2.vi" "Vel LDA2 Non Coincident"() -> (w584:dbl[])
                  n219 = global read "LDA_meas_global_2.vi" "Arrival times LDA2"() -> (w585:dbl[])
                  n220 = global read "LDA_meas_global_2.vi" "Transit times LDA2"() -> (w586:dbl[])
                }
              }
              n221 = Bundle By Name(cluster=w576, "Eng Values"=w574, "Time (s)"=w573, "Weighting"=w575) -> (w572:T6)
              n222 = call "Remove_LDA_Spikes.vi"("Current Block Number"=w568, "Analaysis info Cluster"=w570, "Time Trace In"=w572) -> ("Analaysis info Cluster Out"=w569:T3, "Time trace Out"=w571:T6)  [unwired: 1 in]
            }
          }
        }
        n223 = And(x=w539, y=w540) -> (x .and. y?=w538:bool)
        n224 = global write "Meas_global.vi" "Analysis Info cluster"(w536) -> ()
        n225 = global write "Meas_global.vi" "Time Trace"(w532) -> ()
      }
      frame 15 {
        w596 = FALSE  # Dialog Box (T)
        n226 = Array Size(array=w590) -> (size(s)=w589:i32[])
        n227 = global read "Meas_global.vi" "Analysis Info cluster"() -> (w605:T3[])
        n228 = Index Array(array=w589, index=1) -> (element=w587:i32)
        n229 = for {
          shift-right: [w617] -> w593
          shift-left: "" -> [w618]
          tunnel: 4 ("Index") -> [w624]
          tunnel: w604 -> [w621]
          tunnel: w587 -> [w616]
          tunnel: w605 -> [w614] mode=indexing
          tunnel: w592 -> [w609]
          i -> [w623]
          n230 = Unbundle By Name(w614) -> ("Inst name"=w613:string)
          n231 = Add(x=w624, y=w623) -> (x+y=w622:i32)
          n232 = Index Array(array=w621, index=w622) -> (element=w611:dbl)
          n233 = Divide(x=w611, y=w609) -> (x/y=w610:dbl)
          n234 = Divide(x=w610, y=w616) -> (x/y=w620:dbl)
          n235 = Greater?(x=w620, y=0.5) -> (0:w612:bool)
          n236 = case shown="True" w612 {
            tunnel: w618 -> [w625 w631]
            tunnel: [w625 w630] -> w617
            tunnel: w610 -> [_ w629]
            tunnel: w616 -> [_ w628]
            tunnel: "%s has an average of %.0f invalid bursts for a block size of %.0f.\n" ("Format String") -> [_ w627]
            tunnel: w613 -> [_ w626]
            frame False {
            }
            frame True {
              n237 = Format Into String(format string=w627, initial string=w631, w626, w629, w628) -> (resulting string=w630:string)  [unwired: 1 in, 1 out]
            }
          }
        }
        n238 = Empty String/Path?(string/path=w593) -> (empty?=w598:bool)
        n239 = Not(x=w598) -> (.not. x?=w599:bool)
        n240 = Bundle By Name(cluster=errorcluster {"status"=FALSE, "code"=0, "source"=""} ("error in (no error)"), "source"=w593, "status"=w599) -> (w595:errorcluster)
        n241 = global read "Meas_global.vi" "Extra Comments"() -> (w600:string)
        n242 = Concatenate Strings(w600, w593) -> (w601:string)
        n243 = global write "Meas_global.vi" "Extra Comments"(w601) -> ()
        n244 = call "EnFlo_Error_Handler.vi"("error in (no error)"=w595, "Error Type"="LDA Invalid Bursts", "Dialog Box (T)"=w596) -> ()  [unwired: 3 out]
      }
    }
  }
  "Sync Index" <- w7
